vi "Write Var Info.vi"(8 "error in":errorcluster, 9 "var info":T1, 10 "name":string, 11 "SharedVariableWrapper in":refnum<class "SharedVariableWrapper.lvclass">) -> (0 "error out":errorcluster, 3 "SharedVariableWrapper out":refnum<class "SharedVariableWrapper.lvclass">)   [LabVIEW 2019, in "SharedVariableWrapper.lvclass"]
uses:
  SharedVariableWrapper.lvclass
  shared variable info.ctl
  SharedVariableWrapper.lvclass/SharedVariableWrapper.ctl
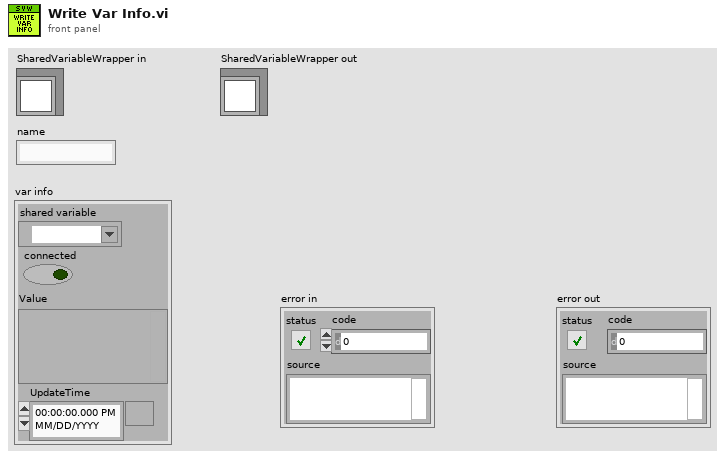
[diagram p1: front panel]
types:
  T1 = typedef "SharedVariableWrapper.lvclass/shared variable info.ctl" = cluster{"shared variable":refnum<k21>, "connected":bool, "Value":variant, "UpdateTime":timestamp}
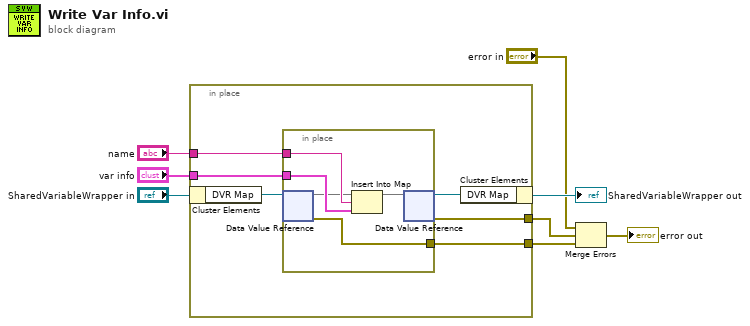
[diagram p0: block diagram]
diagram:
  n1 = in-place {
    in-place-border: "name" -> [w14]
    in-place-border: "var info" -> [w13]
    in-place-border: [w10] -> w4
    in-place-border: [w9] -> w3
    n2 = in-place-cluster #1("SharedVariableWrapper in") -> ("DVR Map"=w12:refnum<data-value>)
    n3 = in-place {
      in-place-border: w14 -> [w19]
      in-place-border: w13 -> [w18]
      in-place-border: [w15] -> w9
      n4 = in-place-dvr #2(w12) -> (w17:map{string, T1}, w15:errorcluster)
      n5 = Insert Into Map(map in=w17, key=w19, value=w18) -> (map out=w16:map{string, T1})  [unwired: 2 out]
      n6 = in-place-dvr #2(w16) -> (w11:refnum<data-value>, w10:errorcluster)
    }
    n7 = in-place-cluster #1("DVR Map"=w11) -> (→"SharedVariableWrapper out":refnum<class "SharedVariableWrapper.lvclass">)
  }
  n8 = Merge Errors("error in", w4, w3) -> (→"error out":errorcluster)
